vi "collide.vi"(4 "Direction in":cluster{"x_dir":i32, "y_dir":i32}, 6 "Brick Ref":refnum<vi>, 7 "Ball Ref":refnum<vi>) -> (0 "Direction":cluster{"x_dir":i32, "y_dir":i32}, 2 "Hit":bool, 3 "Brick out":refnum<vi>)   [LabVIEW 8.6]
uses:
  VI_Control/Brick Pos Ctrl.ctl
  VI_Control/Ball Center Ctrl.ctl
panel:
  in  "Brick":bool
  in  "Ball":bool
  out "Hit_V":bool
  out "Hit_H":bool
  out "y2 to btm":dbl
  out "Ball Center":T1
  out "Pos: Brick":T2
  out "y1 to top":dbl
  out "Hit Corner":bool
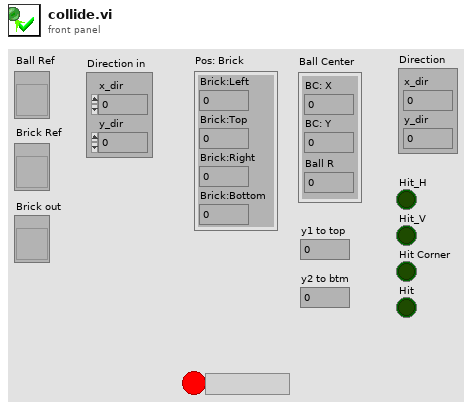
[diagram p1: front panel]
types:
  T1 = typedef "Ball Center Ctrl.ctl" = cluster{"BC: X":i32, "BC: Y":i32, "Ball R":i32}
  T2 = typedef "Brick Pos Ctrl.ctl" = cluster{"Brick:Left":i32, "Brick:Top":i32, "Brick:Right":i32, "Brick:Bottom":i32}
  T3 = cluster{"Brick:Left":i32, "Brick:Top":i32, "Brick:Right":i32, "Brick:Bottom":i32}
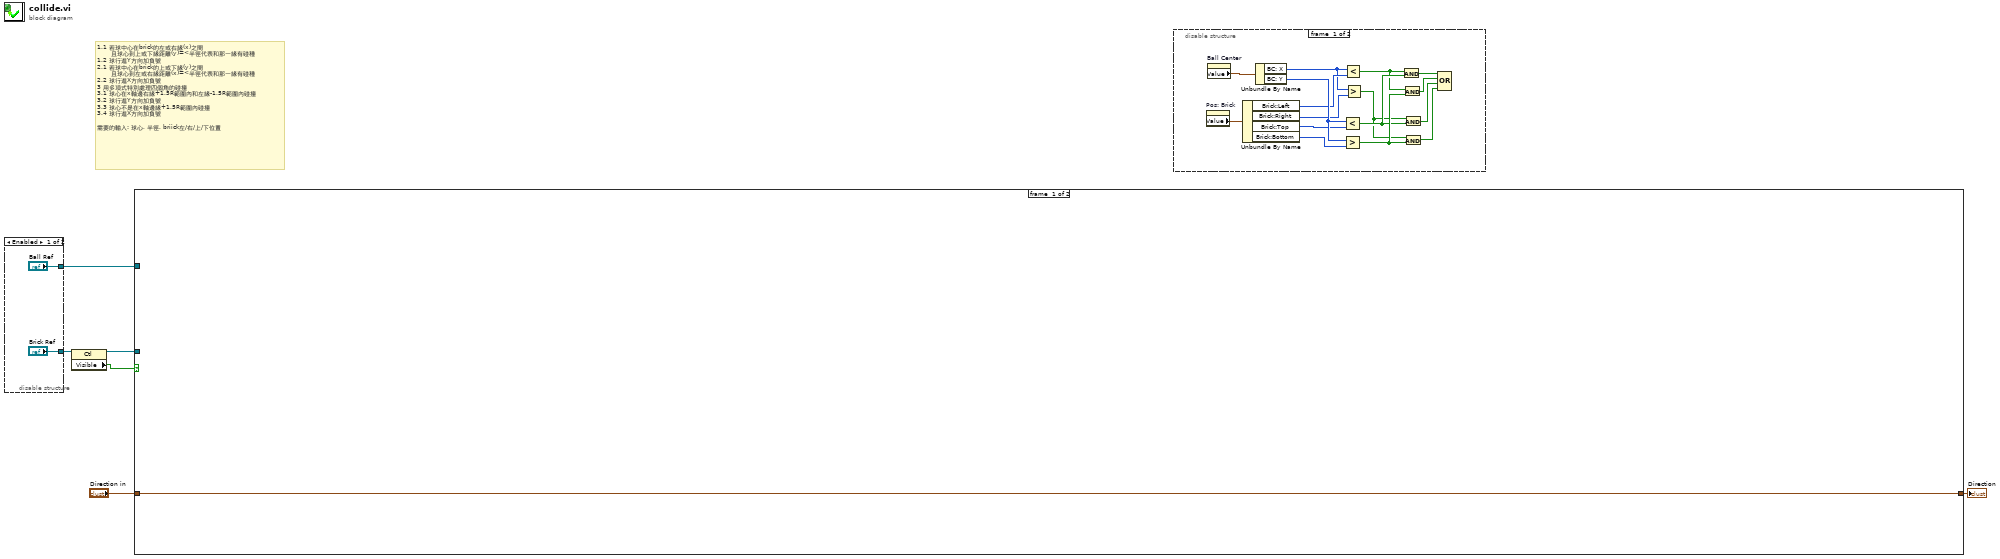
[diagram p0: block diagram]
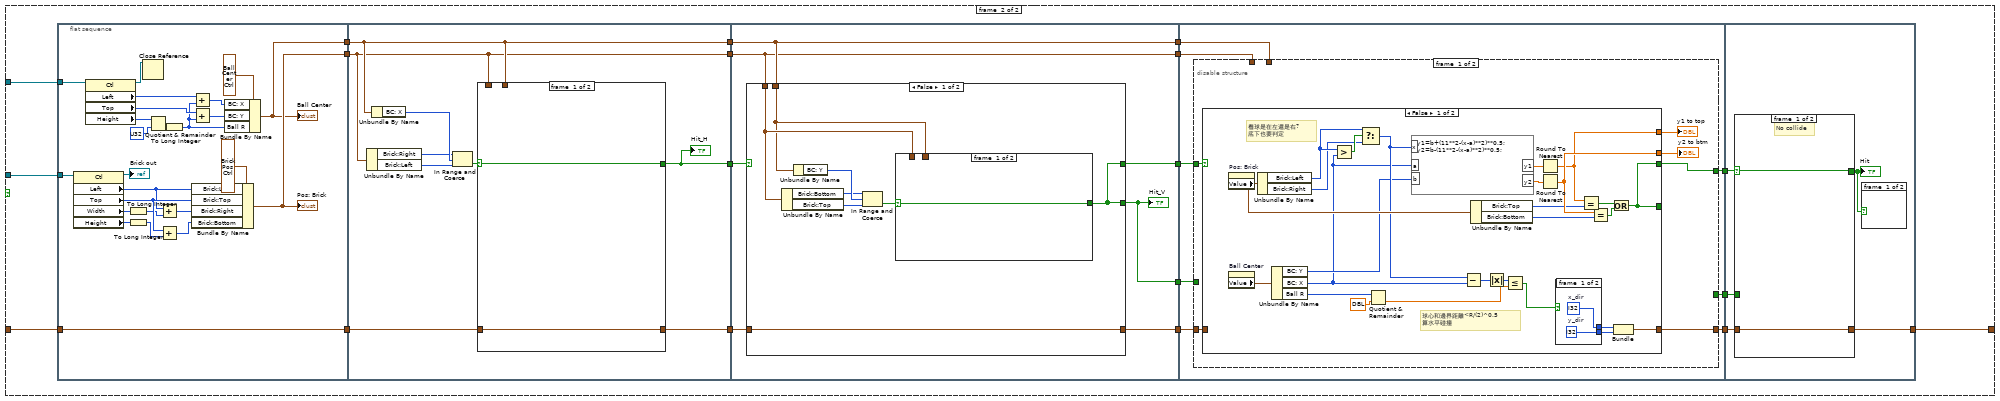
[diagram p2: hidden frame]
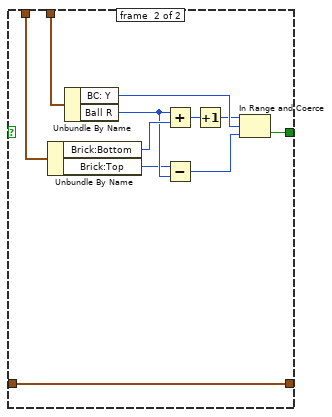
[diagram p3: hidden frame]
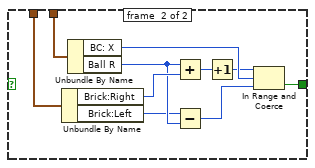
[diagram p4: hidden frame]
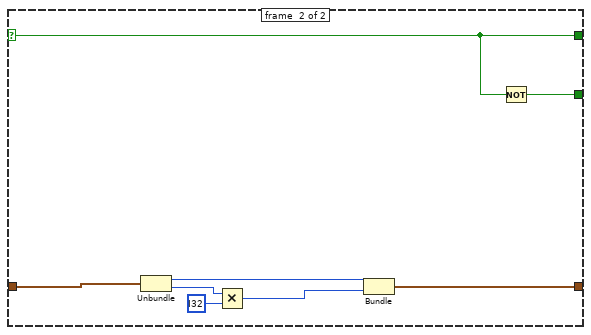
[diagram p5: hidden frame]
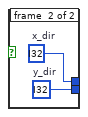
[diagram p6: hidden frame]
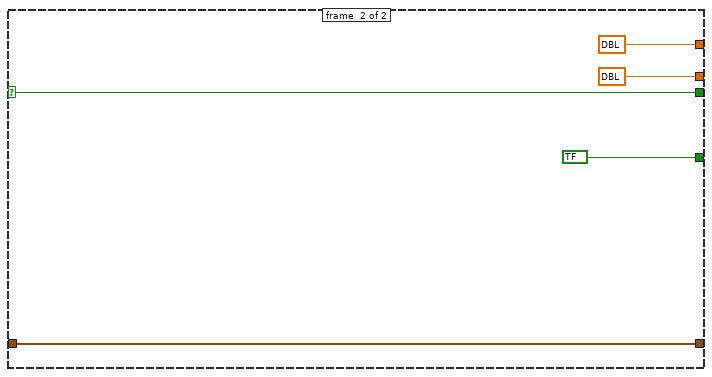
[diagram p7: hidden frame]
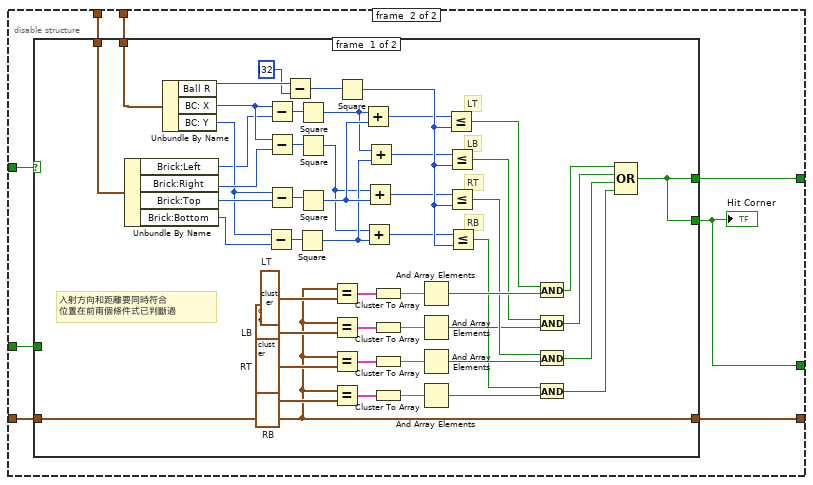
[diagram p8: hidden frame]
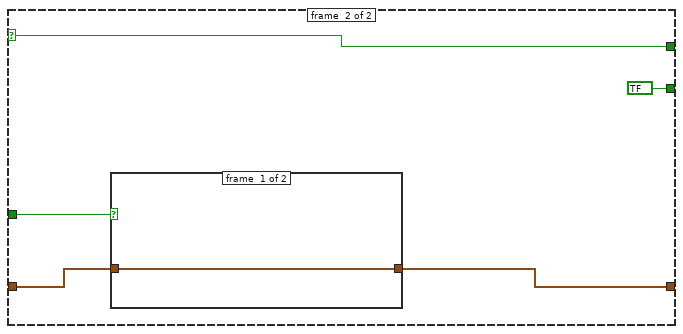
[diagram p9: hidden frame]
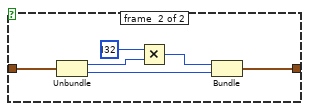
[diagram p10: hidden frame]
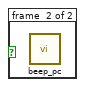
[diagram p11: hidden frame]
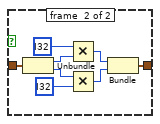
[diagram p13: hidden frame]
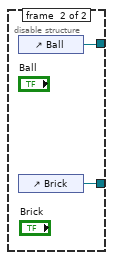
[diagram p14: hidden frame]
diagram:
  # "1.1 若球中心在brick的左或右緣(x)之間\n       且球心到上或下緣距離(y)=<半徑代表和那一緣有碰種\n1.2 球行進Y方向加負號\n2.1 若球中心在brick的上或下緣(y)之間\n       且球心到左或右緣距離(x)=<半徑代表和那一緣有碰種\n2.2 球行進X方向加負號\n3 用多項式特別處理四個角的碰撞\n3.1 球心在x軸邊右緣+1.5R範圍內和左緣-1.5R範圍內碰撞\n3.2 球行進Y方向加負號\n3.3 球心不是在x軸邊緣+1.5R範圍內碰撞\n3.4 球行進X方向加負號\n\n需要的輸入: 球心, 半徑, briick左/右/上/下位置"
  n1 = disable-structure shown="Enabled" {
    disable-tunnel: ["Brick Ref" w10] -> w5
    disable-tunnel: ["Ball Ref" w9] -> w6
    frame #0 {
    }
    frame #1 {
      n2 = control-ref of="Ball"() -> (w9:refnum<vi>)
      n3 = control-ref of="Brick"() -> (w10:refnum<vi>)
    }
  }
  n4 = property class="Ctl"(reference=w5) -> (reference out=w4:refnum<vi>, "Visible"=w3:bool)  [unwired: 1 in, 1 out]
  n5 = case shown="True" w3 {
    tunnel: w6 -> [_ w20]
    tunnel: w4 -> [_ w19]
    tunnel: "Direction in" -> [w11 w13]
    tunnel: [w11 w12] -> w1
    frame #0 {
    }
    frame #1 {
      n6 = flat-sequence {
        tunnel: w20 -> [w37]
        tunnel: w19 -> [w36]
        tunnel: [w33] -> w30
        tunnel: [w31] -> w29
        tunnel: [w35] -> w28
        tunnel: w13 -> [w33]
        tunnel: [w64] -> w27
        tunnel: [w63] -> w26
        tunnel: [w61] -> w18
        tunnel: [w60] -> w17
        tunnel: w28 -> [w60]
        tunnel: w29 -> [w61]
        tunnel: w30 -> [w62]
        tunnel: [w81] -> w25
        tunnel: [w84] -> w24
        tunnel: [w83] -> w16
        tunnel: [w82] -> w15
        tunnel: w17 -> [w82]
        tunnel: w18 -> [w83]
        tunnel: w26 -> [w79]
        tunnel: w27 -> [w80]
        tunnel: [w78] -> w14
        tunnel: w25 -> [w119]
        tunnel: [w117] -> w23
        tunnel: [w116] -> w22
        tunnel: w24 -> [w115]
        tunnel: [w114] -> w21
        tunnel: w16 -> [w113]
        tunnel: w15 -> [w112]
        tunnel: w14 -> [w118]
        tunnel: w23 -> [w235]
        tunnel: w22 -> [w234]
        tunnel: w21 -> [w233]
        tunnel: [w232] -> w12
        frame #0 {
          n7 = property class="Ctl"(reference=w36) -> (reference out=→"Brick out":refnum<vi>, "Left"=w51:i32, "Top"=w52:i32, "Width"=w43:u32, "Height"=w46:u32)  [unwired: 1 in, 1 out]
          n8 = property class="Ctl"(reference=w37) -> (reference out=w32:refnum<vi>, "Left"=w54:i32, "Top"=w53:i32, "Height"=w41:u32)  [unwired: 1 in, 1 out]
          n9 = To Long Integer(number=w43) -> (32bit integer=w42:i32)
          n10 = To Long Integer(number=w46) -> (32bit integer=w45:i32)
          n11 = Close Reference(reference=w32) -> ()  [unwired: 1 in, 1 out]
          n12 = Quotient & Remainder(x=w41, y=u32 ?) -> (floor(x/y)=w40:u32)  [unwired: 1 out]
          n13 = Add(x=w51, y=w42) -> (x+y=w44:i32)
          n14 = Add(x=w52, y=w45) -> (x+y=w47:i32)
          n15 = To Long Integer(number=w40) -> (32bit integer=w39:i32)
          n16 = Bundle By Name(cluster=T2 ? ("Pos: Brick"), "Brick:Left"=w51, "Brick:Top"=w52, "Brick:Right"=w44, "Brick:Bottom"=w47) -> (w35:T2)
          "Pos: Brick" <- w35
          n17 = Add(x=w54, y=w39) -> (x+y=w49:i32)
          n18 = Add(x=w53, y=w39) -> (x+y=w48:i32)
          n19 = Bundle By Name(cluster=T1 ? ("Ball Center 3"), "BC: X"=w49, "BC: Y"=w48, "Ball R"=w39) -> (w31:T1)
          "Ball Center" <- w31
        }
        frame #1 {
          n20 = Unbundle By Name(w60) -> ("Brick:Right"=w56:i32, "Brick:Left"=w58:i32)
          n21 = Unbundle By Name(w61) -> ("BC: X"=w59:i32)
          n22 = In Range and Coerce(upper limit=w56, x=w59, lower limit=w58) -> (In Range?=w57:bool)  [unwired: 1 out]
          n23 = case shown="True" w57 {
            selector: w57 -> [w66 _]
            tunnel: [w66 w71] -> w64
            tunnel: [w65 w77] -> w63
            tunnel: w62 -> [w65 w77]
            tunnel: w61 -> [_ w76]
            tunnel: w60 -> [_ w75]
            frame #0 {
            }
            frame #1 {
              n24 = Unbundle By Name(w75) -> ("Brick:Bottom"=w74:i32, "Brick:Top"=w69:i32)
              n25 = Unbundle By Name(w76) -> ("BC: Y"=w72:i32, "Ball R"=w70:i32)
              n26 = Add(x=w70, y=w74) -> (x+y=w68:i32)
              n27 = Subtract(x=w69, y=w70) -> (x-y=w73:i32)
              n28 = Increment(x=w68) -> (x+1=w67:i32)
              n29 = In Range and Coerce(upper limit=w67, x=w72, lower limit=w73) -> (In Range?=w71:bool)  [unwired: 1 out]
            }
          }
          "Hit_H" <- w64
        }
        frame #2 {
          n30 = case shown="False" w80 {
            selector: w80 -> [_ w105]
            tunnel: [w89 w105] -> w81
            tunnel: [w92 w106] -> w78
            tunnel: [w89 w104] -> w84
            tunnel: w79 -> [w92 w111]
            tunnel: w83 -> [w90 _]
            tunnel: w82 -> [w91 _]
            frame #0 {
              n31 = Unbundle By Name(w91) -> ("Brick:Bottom"=w85:i32, "Brick:Top"=w86:i32)
              n32 = Unbundle By Name(w90) -> ("BC: Y"=w88:i32)
              n33 = In Range and Coerce(upper limit=w85, x=w88, lower limit=w86) -> (In Range?=w87:bool)  [unwired: 1 out]
              n34 = case shown="True" w87 {
                selector: w87 -> [w93 _]
                tunnel: w90 -> [_ w103]
                tunnel: w91 -> [_ w102]
                tunnel: [w93 w98] -> w89
                frame #0 {
                }
                frame #1 {
                  n35 = Unbundle By Name(w102) -> ("Brick:Right"=w101:i32, "Brick:Left"=w96:i32)
                  n36 = Unbundle By Name(w103) -> ("BC: X"=w100:i32, "Ball R"=w97:i32)
                  n37 = Add(x=w97, y=w101) -> (x+y=w95:i32)
                  n38 = Subtract(x=w96, y=w97) -> (x-y=w99:i32)
                  n39 = Increment(x=w95) -> (x+1=w94:i32)
                  n40 = In Range and Coerce(upper limit=w94, x=w100, lower limit=w99) -> (In Range?=w98:bool)  [unwired: 1 out]
                }
              }
            }
            frame #1 {
              n41 = Unbundle(w111) -> ("x_dir"=w107:i32, "y_dir"=w110:i32)
              n42 = Multiply(x=w110, y=i32 ?) -> (x*y=w108:i32)
              n43 = Bundle("x_dir"=w107, w108) -> (w106:cluster{"x_dir":i32, i32})  [unwired: 1 in]
              n44 = Not(x=w105) -> (.not. x?=w104:bool)
            }
          }
          "Hit_V" <- w84
        }
        frame #3 {
          n45 = disable-structure shown="Enabled" {
            disable-tunnel: w119 -> [w125 w168]
            disable-tunnel: w118 -> [w124 w165]
            disable-tunnel: [w123 w167] -> w117
            disable-tunnel: [w122 w166] -> w116
            disable-tunnel: w115 -> [_ w164]
            disable-tunnel: [_ w163] -> w114
            disable-tunnel: w113 -> [_ w162]
            disable-tunnel: w112 -> [_ w161]
            frame #0 {
              n46 = case shown="False" w125 {
                selector: w125 -> [_ w159]
                tunnel: w124 -> [_ w160]
                tunnel: [w142 w160] -> w122
                tunnel: [w141 w159] -> w123
                tunnel: [w141 bool ?] -> _
                tunnel: [w139 dbl ?] -> w121
                tunnel: [w138 dbl ?] -> w120
                frame #0 {
                  # "球心和邊界距離<R/(2)^0.5\n算水平碰撞"
                  # "看球是在左還是右?\n底下也要判定"
                  n47 = property on="Pos: Brick" class="Clust (strict)"() -> ("Value"=w134:T3)  [unwired: 2 in, 2 out]
                  n48 = property on="Ball Center" class="Clust (strict)"() -> ("Value"=w135:cluster{"BC: X":i32, "BC: Y":i32, "Ball R":i32})  [unwired: 2 in, 2 out]
                  n49 = Unbundle By Name(w134) -> ("Brick:Left"=w131:i32, "Brick:Right"=w130:i32)
                  n50 = Unbundle By Name(w135) -> ("BC: Y"=w127:i32, "BC: X"=w126:i32, "Ball R"=w146:i32)
                  n51 = Greater?(x=w131, y=w126) -> (0:w140:bool)
                  n52 = Select(t=w131, s=w140, f=w130) -> (s? t:f=w128:i32)
                  n53 = Quotient & Remainder(x=w146, y=dbl ?) -> (floor(x/y)=w145:dbl)  [unwired: 1 out]
                  n54 = formula code="y1=b+(11**2-(x-a)**2)**0.5;\ny2=b-(11**2-(x-a)**2)**0.5;"("a"=w126, "b"=w127, "x"=w128) -> ("y1"=w150:dbl, "y2"=w151:dbl)
                  n55 = Subtract(x=w128, y=w126) -> (x-y=w132:i32)
                  n56 = Unbundle By Name(w134) -> ("Brick:Top"=w137:i32, "Brick:Bottom"=w136:i32)
                  n57 = Absolute Value(x=w132) -> (abs(x)=w133:i32)
                  n58 = Less Or Equal?(x=w133, y=w145) -> (x <= y?=w129:bool)
                  n59 = Round To Nearest(number=w150) -> (nearest integer value=w138:dbl)
                  n60 = Round To Nearest(number=w151) -> (nearest integer value=w139:dbl)
                  n61 = case shown="True" w129 {
                    tunnel: [w152 w155] -> w144
                    tunnel: [w153 w154] -> w143
                    frame #0 {
                      w153 = i32 ?  # y_dir
                      w152 = i32 ?  # x_dir
                    }
                    frame #1 {
                      w154 = i32 ?  # y_dir
                      w155 = i32 ?  # x_dir
                    }
                  }
                  n62 = Equal?(x=w138, y=w137) -> (x = y?=w149:bool)
                  n63 = Equal?(x=w139, y=w136) -> (x = y?=w148:bool)
                  n64 = Or(x=w149, y=w148) -> (x .or. y?=w141:bool)
                  n65 = Bundle("x_dir"=w144, "y_dir"=w143) -> (w142:cluster{"x_dir":i32, "y_dir":i32})  [unwired: 1 in]
                }
                frame #1 {
                }
              }
              "y2 to btm" <- w121
              "y1 to top" <- w120
            }
            frame #1 {
              n66 = case shown="True" w168 {
                selector: w168 -> [_ w223]
                tunnel: [w202 w223] -> w167
                tunnel: [w192 w220] -> w166
                tunnel: w165 -> [w192 w221]
                tunnel: [w202 bool ?] -> w163
                tunnel: w164 -> [_ w219]
                tunnel: w162 -> [w170 _]
                tunnel: w161 -> [w169 _]
                frame #0 {
                  w195 = cluster{i32, i32} ?  # RB
                  w193 = cluster{i32, i32} ?  # LB
                  w211 = cluster{i32, i32} ?  # RT
                  w200 = cluster{i32, i32} ?  # LT
                  # "RB"
                  # "LB"
                  # "入射方向和距離要同時符合\n位置在前兩個條件式已判斷過"
                  # "RT"
                  # "LT"
                  n67 = Unbundle By Name(w169) -> ("Brick:Left"=w185:i32, "Brick:Right"=w217:i32, "Brick:Top"=w216:i32, "Brick:Bottom"=w184:i32)
                  n68 = Unbundle By Name(w170) -> ("Ball R"=w199:i32, "BC: X"=w218:i32, "BC: Y"=w186:i32)
                  n69 = Subtract(x=w186, y=w184) -> (x-y=w187:i32)
                  n70 = Subtract(x=w218, y=w185) -> (x-y=w215:i32)
                  n71 = Subtract(x=w218, y=w217) -> (x-y=w213:i32)
                  n72 = Subtract(x=w186, y=w216) -> (x-y=w214:i32)
                  n73 = Subtract(x=w199, y=i32 ?) -> (x-y=w176:i32)
                  n74 = Square(x=w187) -> (x^2=w183:i32)
                  n75 = Square(x=w215) -> (x^2=w182:i32)
                  n76 = Square(x=w213) -> (x^2=w180:i32)
                  n77 = Square(x=w214) -> (x^2=w212:i32)
                  n78 = Equal?(x=w192, y=w200) -> (x = y?=w210:cluster{bool, bool})
                  n79 = Equal?(x=w192, y=w193) -> (x = y?=w191:cluster{bool, bool})
                  n80 = Equal?(x=w192, y=w211) -> (x = y?=w209:cluster{bool, bool})
                  n81 = Equal?(x=w192, y=w195) -> (x = y?=w194:cluster{bool, bool})
                  n82 = Square(x=w176) -> (x^2=w175:i32)
                  n83 = Add(x=w182, y=w212) -> (x+y=w174:i32)
                  n84 = Add(x=w180, y=w183) -> (x+y=w171:i32)
                  n85 = Add(x=w180, y=w212) -> (x+y=w172:i32)
                  n86 = Add(x=w182, y=w183) -> (x+y=w173:i32)
                  n87 = Cluster To Array(cluster=w210) -> (array=w208:bool[])
                  n88 = Cluster To Array(cluster=w191) -> (array=w197:bool[])
                  n89 = Cluster To Array(cluster=w209) -> (array=w207:bool[])
                  n90 = Cluster To Array(cluster=w194) -> (array=w196:bool[])
                  n91 = And Array Elements(Boolean array=w208) -> (logical AND=w206:bool)
                  n92 = And Array Elements(Boolean array=w197) -> (logical AND=w189:bool)
                  n93 = And Array Elements(Boolean array=w207) -> (logical AND=w205:bool)
                  n94 = And Array Elements(Boolean array=w196) -> (logical AND=w190:bool)
                  n95 = Less Or Equal?(x=w174, y=w175) -> (x <= y?=w203:bool)
                  n96 = Less Or Equal?(x=w173, y=w175) -> (x <= y?=w177:bool)
                  n97 = Less Or Equal?(x=w172, y=w175) -> (x <= y?=w204:bool)
                  n98 = Less Or Equal?(x=w171, y=w175) -> (x <= y?=w181:bool)
                  n99 = And(x=w203, y=w206) -> (x .and. y?=w188:bool)
                  n100 = And(x=w177, y=w189) -> (x .and. y?=w178:bool)
                  n101 = And(x=w204, y=w205) -> (x .and. y?=w201:bool)
                  n102 = And(x=w181, y=w190) -> (x .and. y?=w179:bool)
                  n103 = Compound Arithmetic op=OR(w188, w178, w201, w179) -> (w202:bool)
                }
                frame #1 {
                  n104 = case shown="True" w219 {
                    tunnel: w221 -> [w224 w226]
                    tunnel: [w224 w225] -> w220
                    frame #0 {
                    }
                    frame #1 {
                      n105 = Unbundle(w226) -> ("x_dir"=w228:i32, "y_dir"=w227:i32)
                      n106 = Multiply(x=i32 ? ("y"), y=w228) -> (x*y=w230:i32)
                      n107 = Bundle(w230, "y_dir"=w227) -> (w225:cluster{i32, "y_dir":i32})  [unwired: 1 in]
                    }
                  }
                }
              }
              "Hit Corner" <- w163
            }
          }
        }
        frame #4 {
          n108 = case shown="True" w235 {
            selector: w235 -> [w237 w241]
            tunnel: w234 -> [w236 w239]
            tunnel: [w236 w240] -> w232
            tunnel: [w237 w241] -> w231
            tunnel: w233 -> [_ w238]
            frame #0 {
              # "No collide"
            }
            frame #1 {
              n109 = case shown="True" w238 {
                tunnel: [w242 w244] -> w240
                tunnel: w239 -> [w242 w243]
                frame #0 {
                }
                frame #1 {
                  n110 = Unbundle(w243) -> ("x_dir"=w245:i32, "y_dir"=w249:i32)
                  n111 = Multiply(x=i32 ? ("y"), y=w245) -> (x*y=w247:i32)
                  n112 = Multiply(x=w249, y=i32 ?) -> (x*y=w248:i32)
                  n113 = Bundle(w247, w248) -> (w244:cluster{i32, i32})  [unwired: 1 in]
                }
              }
            }
          }
          "Hit" <- w231
          n114 = case shown="True" w231 {
            frame #0 {
            }
            frame #1 {
              n115 = call "beep_pc.vi"() -> ()  [unwired: 4 in, 1 out]
            }
          }
        }
      }
    }
  }
  "Direction" <- w1
  n116 = disable-structure shown="Enabled" {
    frame #0 {
      n117 = property on="Pos: Brick" class="Clust (strict)"() -> ("Value"=w252:T3)  [unwired: 2 in, 2 out]
      n118 = property on="Ball Center" class="Clust (strict)"() -> ("Value"=w251:cluster{"BC: X":i32, "BC: Y":i32, "Ball R":i32})  [unwired: 2 in, 2 out]
      n119 = Unbundle By Name(w252) -> ("Brick:Left"=w254:i32, "Brick:Right"=w255:i32, "Brick:Top"=w256:i32, "Brick:Bottom"=w257:i32)
      n120 = Unbundle By Name(w251) -> ("BC: X"=w253:i32, "BC: Y"=w258:i32)
      n121 = Less?(x=w258, y=w256) -> (x < y?=w261:bool)
      n122 = Greater?(x=w258, y=w257) -> (0:w262:bool)
      n123 = Less?(x=w253, y=w254) -> (x < y?=w259:bool)
      n124 = Greater?(x=w253, y=w255) -> (0:w260:bool)
      n125 = And(x=w259, y=w261) -> (x .and. y?=w263:bool)
      n126 = And(x=w259, y=w262) -> (x .and. y?=w264:bool)
      n127 = And(x=w260, y=w261) -> (x .and. y?=w265:bool)
      n128 = And(x=w260, y=w262) -> (x .and. y?=w266:bool)
      n129 = Compound Arithmetic op=OR(w263, w264, w265, w266) -> ()  [unwired: 1 out]
    }
    frame #1 {
    }
  }
